vi "Create.vi"(8 "error in (no error)":errorcluster, 10 "File name (exclude extension)":string, 11 "Folder (create file inside this folder)":path) -> (0 "error out":errorcluster, 3 "Log file path":path)   [LabVIEW 2018, in "text_file.lvlib"]
uses:
  text_file.lvlib
  private_data (library_variable).vi
panel:
  # "Development\ncontrols/indicators useful for development and testing, but which are not outputs of the VI"
  # "Input\nInputs to the VI"
  # "Output\nOutputs of the VI"
  # "Description\n\nBlank VI with error handling case. \n\nSummarize the use of this VI in this space."
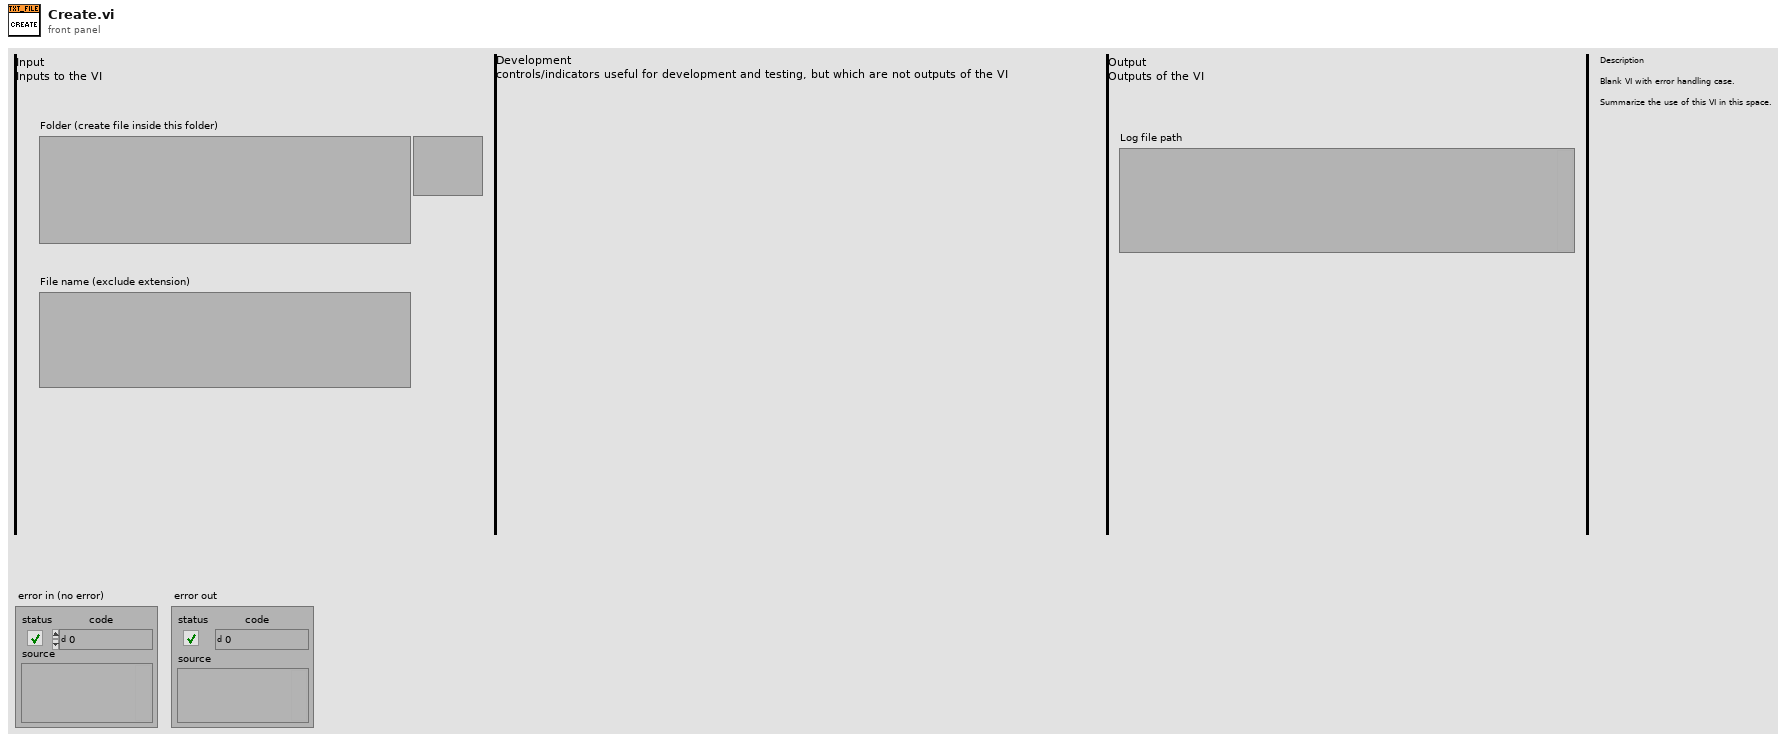
[diagram p1: front panel]
types:
  T1 = enum16{"open", "replace", "create", "open or create", "replace or create", "replace or create with confirmation"}
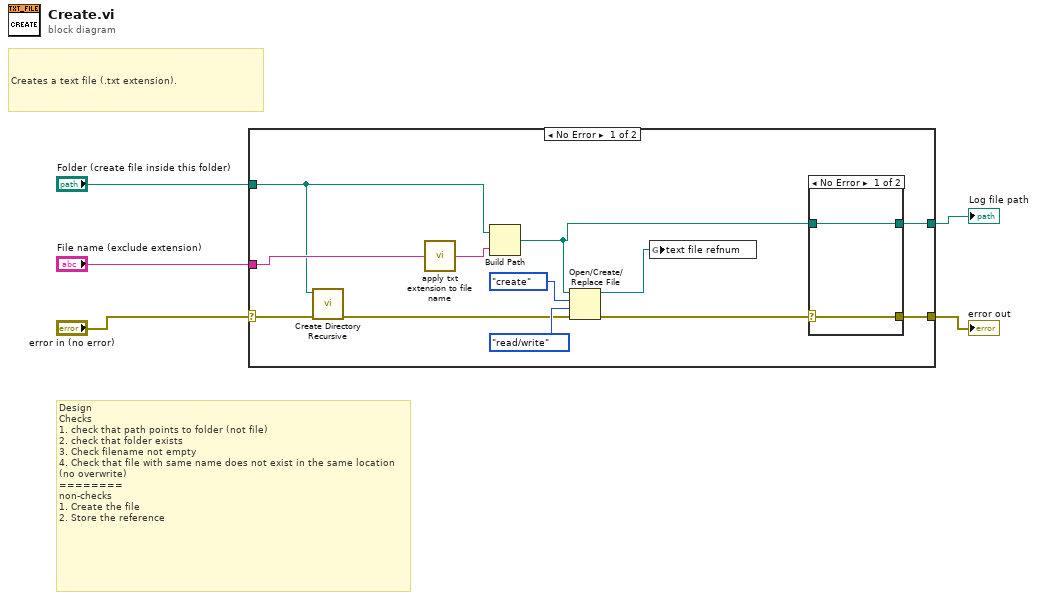
[diagram p0: block diagram]
diagram:
  # "Design\nChecks\n1. check that path points to folder (not file)\n2. check that folder exists\n3. Check filename not empty\n4. Check that file with same name does not exist in the same location (no overwrite)\n========\nnon-checks\n1. Create the file\n2. Store the reference"
  # "Creates a text file (.txt extension)."
  n1 = case shown="No Error" "error in (no error)" {
    selector: "error in (no error)" -> [w11 w21]
    tunnel: [w8 w21] -> w4
    tunnel: "Folder (create file inside this folder)" -> [w9 _]
    tunnel: "File name (exclude extension)" -> [w16 _]
    tunnel: [w7 _] -> w1
    frame No Error {
      n2 = call <vilib>:"Create Directory Recursive.vi"("error in (no error)"=w11, "directory"=w9) -> ("error out"=w10:errorcluster)  [unwired: 3 in, 2 out]
      n3 = call "apply txt extension to file name.vi"("File name (excluding extension)"=w16) -> ("File name (with .txt extension)"=w12:string)
      n4 = Build Path(base path=w9, name or relative path=w12) -> (appended path=w6:path)
      n5 = Open/Create/Replace File(file path (use dialog)=w6, error in=w10, operation (0:open)=T1."create", access (0:read/write)=enum16{"read/write", "read-only", "write-only"}."read/write") -> (refnum out=w13:refnum<file>, error out=w17:errorcluster)  [unwired: 2 in, 1 out]
      n6 = global write "private_data (library_variable).vi" "text file refnum"(w13) -> ()
      n7 = case shown="No Error" w17 {
        selector: w17 -> [w19 w20]
        tunnel: [w19 w20] -> w8
        tunnel: [w18 _] -> w7
        tunnel: w6 -> [w18 _]
        frame No Error {
        }
        frame Error {
        }
      }
    }
    frame Error {
    }
  }
  "error out" <- w4
  "Log file path" <- w1
